vi "_save_cs_string.vi"(7 "FileName":string="SingleCh_", 11 "Array":string[][](array[string])) -> (3 "FileName":string)   [LabVIEW 2023]
uses:
  <vilib>/Utility/file.llb/Write Delimited Spreadsheet (string).vi
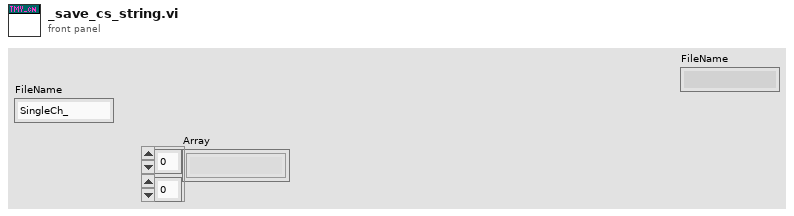
[diagram p1: front panel]
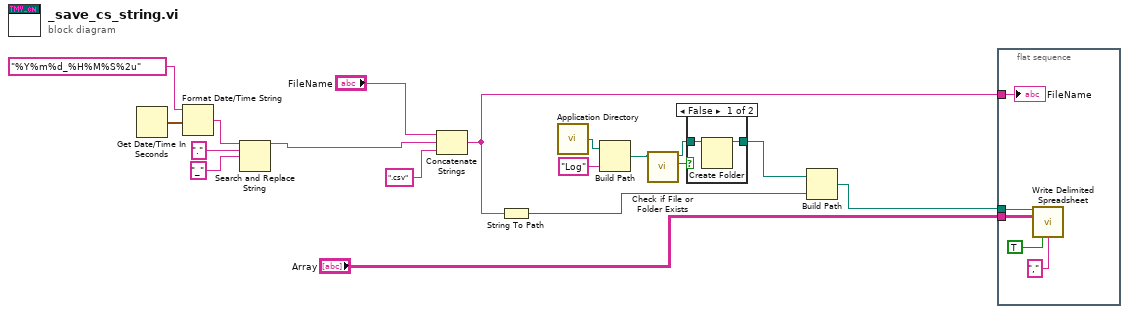
[diagram p0: block diagram]
diagram:
  n1 = Get Date/Time In Seconds() -> (seconds since 1Jan1904=w11:timestamp)
  n2 = Format Date/Time String(time format string (%c)="%Y%m%d_%H%M%S%2u", seconds (now)=w11) -> (date/time string=w9:string)  [unwired: 1 in]
  n3 = Search and Replace String(input string=w9, search string=".", replace string="_") -> (result string=w6:string)  [unwired: 5 in, 3 out]
  n4 = Concatenate Strings("FileName", w6, ".csv" ("delimiter (\\t)")) -> (w15:string)
  n5 = String To Path(string=w15) -> (path=w17:path)
  n6 = call <vilib>:"Application Directory.vi"() -> ("Application Directory"=w14:path)
  n7 = Build Path(base path=w14, name or relative path="Log") -> (appended path=w2:path)
  n8 = call <vilib>:"Check if File or Folder Exists.vi"("path"=w2) -> ("file or folder exists?"=w4:bool, "dup path"=w3:path)  [unwired: 8 in, 1 out]
  n9 = case shown="False" w4 {
    tunnel: w3 -> [w20 w21]
    tunnel: [w19 w21] -> w1
    frame False {
      n10 = Create Folder(path (use dialog)=w20) -> (created path=w19:path)  [unwired: 2 in, 2 out]
    }
    frame True {
    }
  }
  n11 = Build Path(base path=w1, name or relative path=w17) -> (appended path=w5:path)
  n12 = flat-sequence {
    tunnel: w5 -> [w25]
    tunnel: "Array" -> [w24]
    tunnel: w15 -> [w22]
    frame #0 {
      n13 = call-poly <vilib>:"Write Delimited Spreadsheet.vi"("file path (dialog if empty)"=w25, "2D data"=w24, "transpose? (no:F)"=TRUE, "delimiter (\\t)"="," ("delimiter (\\t)")) -> ()  [unwired: 10 in, 2 out]
      "FileName" <- w22
    }
  }
